vi "Set Event (Data).vi"(8 "error in (no error)":errorcluster, 9 "Data":refnum<class "Data.lvclass">, 10 "Event name":string, 11 "Event in":refnum<class "Event.lvclass">) -> (0 "error out":errorcluster, 3 "Event out":refnum<class "Event.lvclass">)   [LabVIEW 2013, in "MDSplus.lvlib" / "Event.lvclass"]
doc: "Issues a new event."
uses:
  <vilib>/MDSplus/Classes/Event_Class/Event.lvclass
  <vilib>/MDSplus/Classes/Data_Class/Data.lvclass
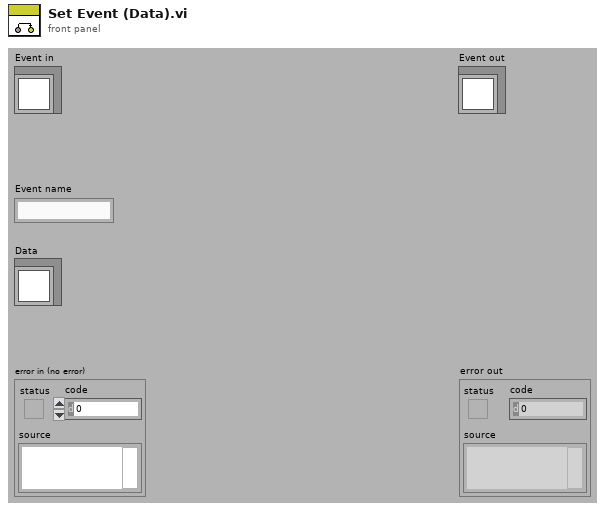
[diagram p1: front panel]
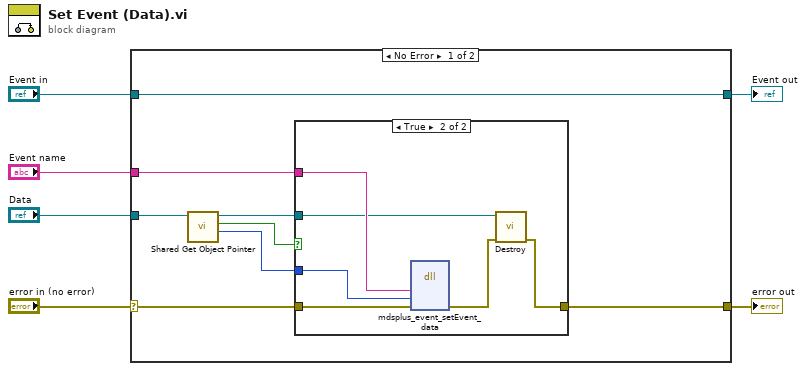
[diagram p0: block diagram]
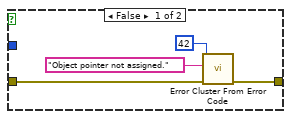
[diagram p2: hidden frame]
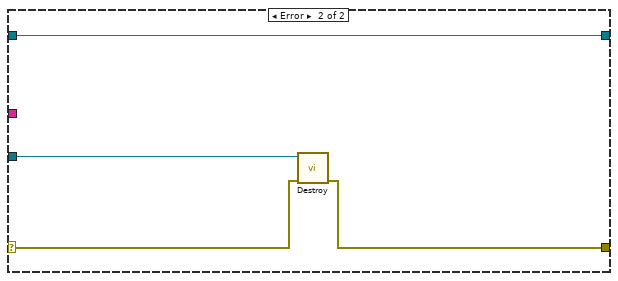
[diagram p3: hidden frame]
diagram:
  n1 = case shown="No Error" "error in (no error)" {
    selector: "error in (no error)" -> [w13 w26]
    tunnel: [w12 w25] -> w5
    tunnel: [w11 w28] -> w4
    tunnel: "Event in" -> [w11 w28]
    tunnel: "Event name" -> [w14 _]
    tunnel: "Data" -> [w10 w27]
    frame No Error {
      n2 = call <vilib>:"Shared Get Object Pointer.vi"("Data in"=w10) -> ("Object Pointer"=w8:i64, "Assigned object pointer?"=w9:bool, "Data out"=w7:refnum<class "Data.lvclass">)  [unwired: 8 in]
      n3 = case shown="True" w9 {
        tunnel: w14 -> [_ w24]
        tunnel: w13 -> [w16 w23]
        tunnel: [w15 w19] -> w12
        tunnel: w8 -> [_ w22]
        tunnel: w7 -> [_ w21]
        frame False {
          n4 = call <vilib>:"Error Cluster From Error Code.vi"("error in (no error)"=w16, "error message (\"\")"="Object pointer not assigned." ("error message (\"\")"), "error code (0)"=42) -> ("error out"=w15:errorcluster)  [unwired: 6 in]
        }
        frame True {
          n5 = dll-call lib="MDSobjectsLVShr" fn="mdsplus_event_setEvent_data"("evNameIn"=w24, "lvDataPtrIn"=w22, "error"=w23) -> ("error"=w20:errorcluster)  [unwired: 6 in, 2 out]
          n6 = call-dynamic "Destroy.vi"("error in (no error)"=w20, "Data in"=w21) -> ("error out"=w19:errorcluster)  [unwired: 9 in]
        }
      }
    }
    frame Error {
      n7 = call-dynamic "Destroy.vi"("error in (no error)"=w26, "Data in"=w27) -> ("error out"=w25:errorcluster)  [unwired: 9 in]
    }
  }
  "error out" <- w5
  "Event out" <- w4
